vi "switchBariumLasersSoftTime.vi"(1 "650":bool=TRUE, 3 "614":bool=TRUE, 4 "1762":bool, 5 "493":bool=TRUE) -> ()   [LabVIEW 2012]
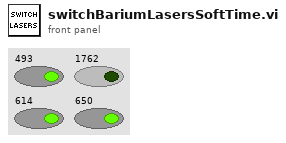
[diagram p1: front panel]
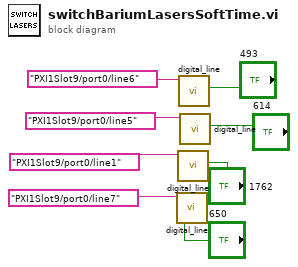
[diagram p0: block diagram]
diagram:
  n1 = call "digital_line.vi"("Boolean"="650", "lines"=tag "PXI1Slot9/port0/line7") -> ()  [unwired: 5 in, 1 out]
  n2 = call "digital_line.vi"("Boolean"="1762", "lines"=tag "PXI1Slot9/port0/line1") -> ()  [unwired: 5 in, 1 out]
  n3 = call "digital_line.vi"("Boolean"="493", "lines"=tag "PXI1Slot9/port0/line6") -> ()  [unwired: 5 in, 1 out]
  n4 = call "digital_line.vi"("Boolean"="614", "lines"=tag "PXI1Slot9/port0/line5") -> ()  [unwired: 5 in, 1 out]
